vi "Part_Image_Skewing.vi"(0 "[IN] Part Image":T1, 1 "[IN] Source Image U16":u16[][](array[numeric]), 2 "[IN] Rows Part":i32, 3 "[IN] Part shift":i32, 5 "[IN] Rows":i32, 9 "[IN] Cols Initial":i32, 11 "error IN":errorcluster, 12 "[IN] tan(theta)":dbl, 14 "[IN] Cols":i32) -> (4 "[OUT] Part Image":T1, 15 "error OUT":errorcluster)   [LabVIEW 2020]
uses:
  <vilib>/vision/Image Controls.llb/IMAQ Image.ctl
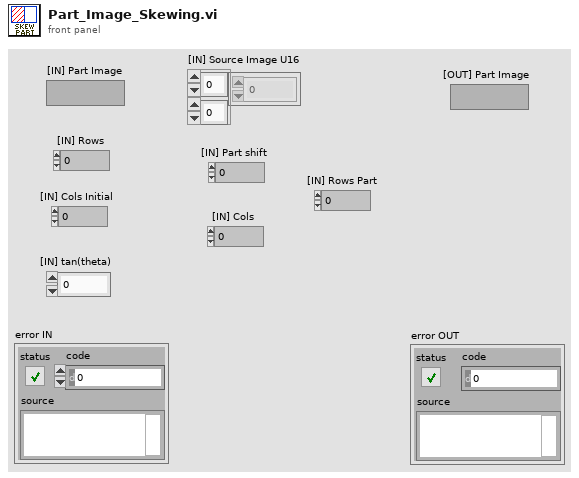
[diagram p1: front panel]
types:
  T1 = typedef "IMAQ Image.ctl" = refnum<image>
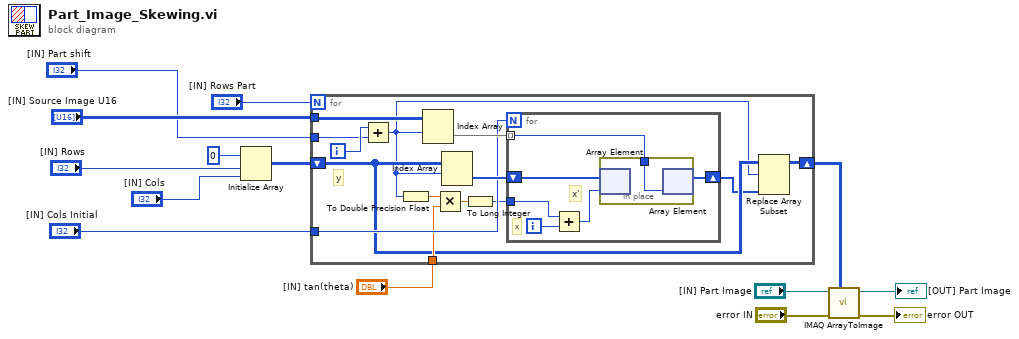
[diagram p0: block diagram]
diagram:
  n1 = Initialize Array(u16 0, "[IN] Rows", "[IN] Cols") -> (w14:u16[][])
  n2 = for {
    N: "[IN] Rows Part" -> [_]
    shift-right: [w19] -> w6
    shift-left: w14 -> [w20]
    tunnel: "[IN] Source Image U16" -> [w27]
    tunnel: "[IN] Cols Initial" -> [w25]
    tunnel: "[IN] tan(theta)" -> [w23]
    tunnel: "[IN] Part shift" -> [w16]
    i -> [w17]
    # "y"
    n3 = Add(x=w17, y=w16) -> (x+y=w15:i32)
    n4 = To Double Precision Float(number=w15) -> (double precision float=w24:dbl)
    n5 = Index Array(array=w27, index (row)=w15) -> (element=w26:u16[])  [unwired: 1 in]
    n6 = Multiply(x=w24, y=w23) -> (x*y=w22:dbl)
    n7 = Index Array(array=w20, index (row)=w15) -> (element=w28:u16[])  [unwired: 1 in]
    n8 = To Long Integer(number=w22) -> (32bit integer=w21:i32)
    n9 = for {
      N: w25 -> [_]
      shift-right: [w30] -> w18
      shift-left: w28 -> [w32]
      tunnel: w26 -> [w29] mode=indexing
      tunnel: w21 -> [w33]
      i -> [w34]
      # "x'"
      # "x"
      n10 = Add(x=w33, y=w34) -> (x+y=w31:i32)
      n11 = in-place {
        in-place-border: w29 -> [w35]
        n12 = in-place-array #1(w32, w31) -> ()  [unwired: 1 out]
        n13 = in-place-array #1(w35) -> (w30:u16[])  [unwired: 1 out]
      }
    }
    n14 = Replace Array Subset(array=w20, new element=w18, index (row)=w15) -> (w19:u16[][])  [unwired: 1 in]
  }
  n15 = call "IMAQ ArrayToImage"("Image Pixels (U16)"=w6, "error in (no error)"="error IN", "Image"="[IN] Part Image") -> ("error out"=→"error OUT":errorcluster, "Image Out"=→"[OUT] Part Image":T1)  [unwired: 7 in]
